vi "Do.vi"(8 "error in":errorcluster, 10 "Actor in":refnum<class "Actor.lvclass">, 11 "Change Laser Gain MSG":refnum<class "Change Laser Gain MSG.lvclass">) -> (0 "error out":errorcluster, 2 "Actor out":refnum<class "Actor.lvclass">)   [LabVIEW 2014, in "eCRDS Library.lvlib" / "Change Laser Gain MSG.lvclass"]
doc: "(<B>Filename</B>: Actor Framework.lvlib:Message.lvclass:Do.vi)\n\nDefines what a message does when it is received by an actor. Generally, a message instructs an actor to invoke one of its methods. By default, this method does nothing. A child class must override it to define behavior. Create a child class by using the Actor Framework Message Maker dialog box."
uses:
  Change Laser Gain MSG.lvclass
  <vilib>/ActorFramework/Actor/Actor.lvclass
  Change Laser Gain MSG.lvclass/Change Laser Gain MSG.ctl
  Instr Actor.lvclass
  Controller/Messages/Update CVT/Update CVT Data.lvclass
  Instr Actor.lvclass/Instr Actor.ctl
  Controller/Messages/Update CVT/Update CVT Data.lvclass/Update CVT Data.ctl
  <vilib>/DAQmx/write.llb/DAQmx Write (Analog 1D DBL NChan 1Samp).vi
  Controller/Messages/Update CVT/Write Data.vi
  Controller/Messages/Update CVT/Write Group.vi
  Controller/Messages/Update CVT/Write tag.vi
  <vilib>/DAQmx/miscellaneous.llb/DAQmx Fill In Error Info.vi
  reusable/Session APIs/Session Log/System Log.lvclass
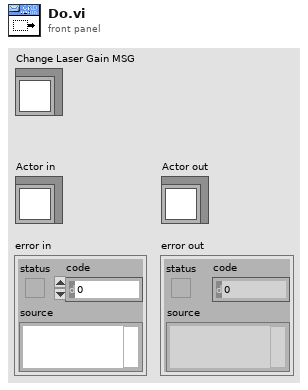
[diagram p1: front panel]
types:
  T1 = typedef "Session - Root.lvclass/Session Handle.ctl" = refnum<data-value>
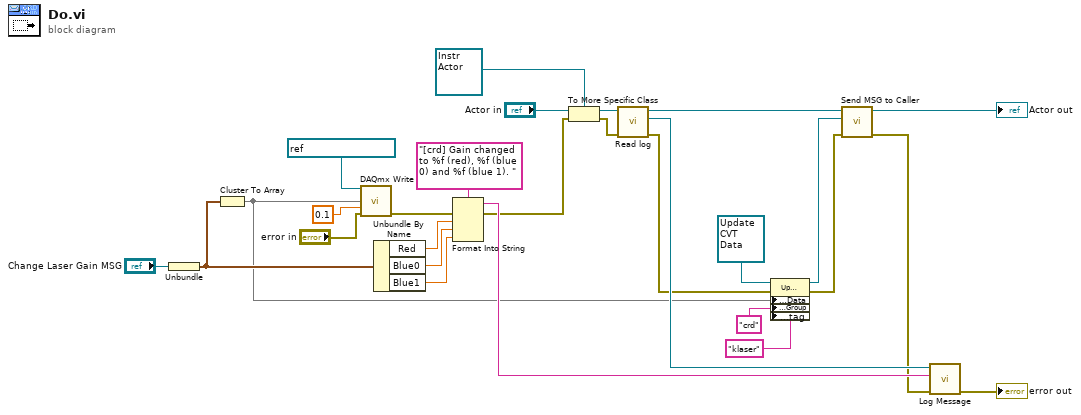
[diagram p0: block diagram]
diagram:
  n1 = Unbundle("Change Laser Gain MSG") -> (w20:cluster{"Red":dbl, "Blue0":dbl, "Blue1":dbl})
  n2 = Cluster To Array(cluster=w20) -> (array=w5:dbl[])
  n3 = call-poly <vilib>:"DAQmx Write.vi"("task/channels in"=refnum<k21> "CRD Laser Gain", "data"=w5, "timeout"=0.1, "error in"="error in") -> ("error out"=w23:errorcluster)  [unwired: 9 in, 2 out]
  n4 = Unbundle By Name(w20) -> ("Red"=w19:dbl, "Blue0"=w18:dbl, "Blue1"=w17:dbl)
  n5 = Format Into String(format string="[crd] Gain changed to %f (red), %f (blue 0) and %f (blue 1). ", error in=w23, w19, w18, w17) -> (resulting string=w22:string, error out=w2:errorcluster)  [unwired: 1 in]
  n6 = To More Specific Class(target class=refnum<class "Instr Actor.lvclass"> refnum ("Instrument Lib:Instr"), reference="Actor in", error in=w2) -> (specific class reference=w15:refnum<class "Instr Actor.lvclass">, error out=w14:errorcluster)
  n7 = call "Read log.vi"("error in (no error)"=w14, "Instr Actor in"=w15) -> ("error out"=w1:errorcluster, "Session Handle"=w13:T1, "Instr Actor out"=w7:refnum<class "Instr Actor.lvclass">)  [unwired: 7 in]
  n8 = property class="Update CVT Data"(reference=refnum<class "Update CVT Data.lvclass"> refnum ("Controller.lvlib:Update CVT Data"), error in=w1, "Accessors:Data"=w5, "Accessors:Group"="crd" ("Group"), "Accessors:tag"="klaser" ("tag")) -> (reference out=w9:refnum<class "Update CVT Data.lvclass">, error out=w8:errorcluster)
  n9 = call "Send MSG to Caller.vi"("error in"=w8, "Message"=w9, "Instr in"=w7) -> ("error out"=w4:errorcluster, "Instr out"=→"Actor out":refnum<class "Instr Actor.lvclass">)  [unwired: 7 in]
  n10 = call "Log Message.vi"("error in"=w4, "MSG In"=w22, "session in"=w13) -> ("error out"=→"error out":errorcluster)  [unwired: 7 in, 1 out]
